vi "test Action Update Set Point-errorCase.vi"() -> ()   [LabVIEW 2018, in "Action Update Set Point.lvclass"]
uses:
  Action Update Set Point.lvclass
  E:/Program Files (x86)/National Instruments/Circuit Design Suite 14.1/LabVIEW 2018/vi.lib/addons/_JKI Toolkits/VI Tester/TestCase.llb/TestCase.lvclass
  <vilib>/addons/_JKI Toolkits/VI Tester/TestCase.llb/TestCase.lvclass
  Libraries/Thermal Chamber Controller_DQMH/Thermal Chamber Controller_DQMH.lvlib
panel:
  out "TestCase out":refnum<class "TestCase.lvclass">
  in  "TestCase in":refnum<class "Action Update Set Point.lvclass">
  out "error out":errorcluster
  in  "error in (no error)":errorcluster
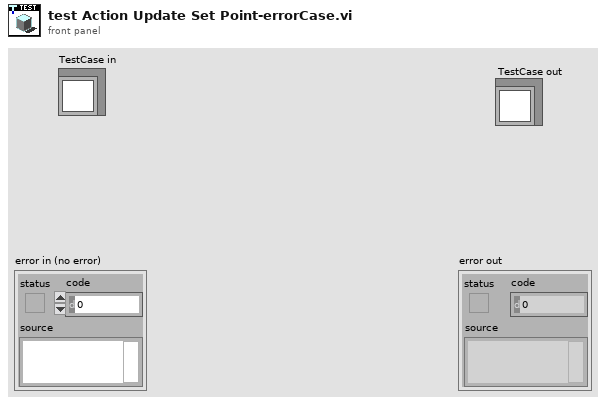
[diagram p1: front panel]
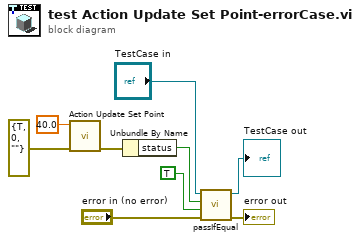
[diagram p0: block diagram]
diagram:
  n1 = call "Action Update Set Point.vi"("error in (no error)"=errorcluster {"status"=TRUE, "code"=0, "source"=""}, "Temperature Set Point"=40.0) -> ("error out"=w4:errorcluster)  [unwired: 9 in]
  n2 = Unbundle By Name(w4) -> ("status"=w1:bool)
  n3 = call-dynamic "passIfEqual.vi"("error in (no error)"="error in (no error)", "y"=TRUE, "x"=w1, "TestCase in"="TestCase in") -> ("error out"=→"error out":errorcluster, "TestCase out"=→"TestCase out":refnum<class "Action Update Set Point.lvclass">)  [unwired: 6 in]
